vi "Read Multiple Data Points.vi"(8 "error in (no error)":errorcluster, 10 "Qty":u32, 11 "34401 in":refnum<class "34401.lvclass">) -> (0 "error out":errorcluster, 2 "Values":dbl[](array[numeric]), 3 "34401 out":refnum<class "34401.lvclass">)   [LabVIEW 2018, in "34401.lvlib" / "34401.lvclass"]
uses:
  34401.lvclass
  34401.lvclass/34401.ctl
  <instrlib>/Agilent 34401/Public/Data/Read (Multiple Points).vi
  <instrlib>/Agilent 34401/Agilent 34401.lvlib
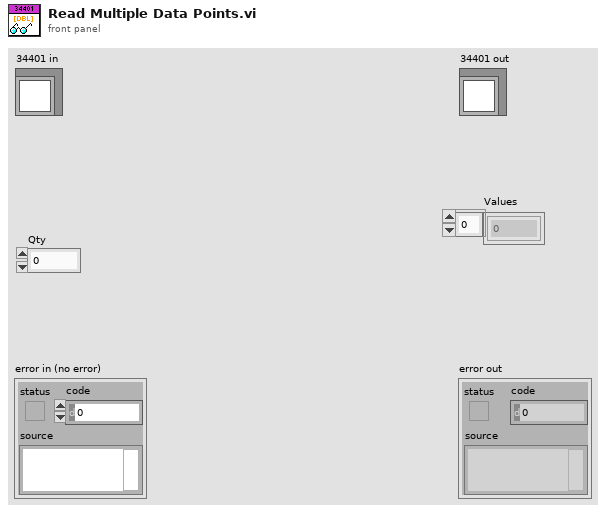
[diagram p1: front panel]
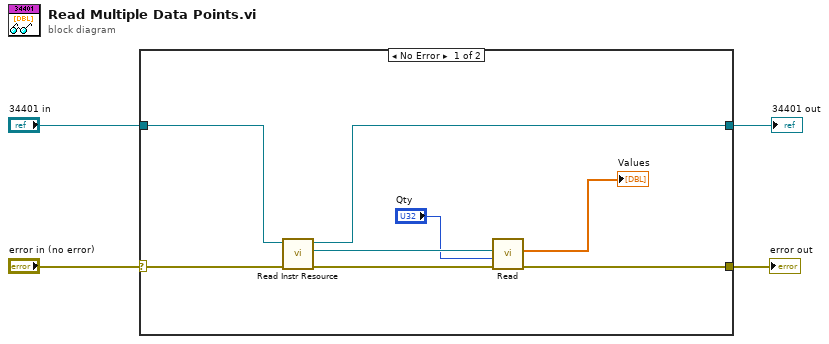
[diagram p0: block diagram]
diagram:
  n1 = case shown="No Error" "error in (no error)" {
    selector: "error in (no error)" -> [w12 w14]
    tunnel: [w5 w14] -> w3
    tunnel: [w7 w13] -> w2
    tunnel: "34401 in" -> [w11 w13]
    frame No Error {
      n2 = call "Read Instr Resource.vi"("error in (no error)"=w12, "34401 in"=w11) -> ("error out"=w10:errorcluster, "Instr Resource"=w9:refnum<visa-resource-name>, "34401 out"=w7:refnum<class "34401.lvclass">)  [unwired: 7 in]
      n3 = call-poly <instrlib>:"Read.vi"("error in (no error)"=w10, "Sample Count (1)"="Qty", "VISA resource name"=w9) -> ("error out"=w5:errorcluster, "Measurements"=→"Values":dbl[])  [unwired: 6 in, 1 out]
    }
    frame Error {
    }
  }
  "error out" <- w3
  "34401 out" <- w2
